vi "TEST adjust Spark Max V PID.vi"(11 "Swerve refs":cluster{"Driver":T1, "Steer":T1, "Encoder":T6}[](array[cluster])) -> ()   [LabVIEW 2023]
uses:
  <vilib>/Rock Robotics/WPI/ThirdParty/REV Robotics/REVLib/Typedef/Spark MAX Smart Motion Parameters.ctl
  <vilib>/Rock Robotics/WPI/MotorControl/WPI_MotorControlDeviceRef.ctl
  <vilib>/Rock Robotics/WPI/MotorControl/WPI_MotorControlType.ctl
  <vilib>/Rock Robotics/SystemInterfaces/DIO/FPGA_DIOPWMChannel.ctl
  <vilib>/Rock Robotics/WPI/PWM/WPI_PWMDeadband.ctl
  <vilib>/Rock Robotics/SystemInterfaces/DIO/FPGA_DIOChannel.ctl
  <vilib>/Rock Robotics/WPI/ThirdParty/Phoenix-LabVIEW/CANCoder/Controls/CTRE_Phoenix_CANcoder_DeviceRef.ctl
  <vilib>/Rock Robotics/WPI/ThirdParty/REV Robotics/REVLib/Typedef/Spark MAX Control Type.ctl
panel:
  out "Sensor Velocity":dbl
  in  "Boolean":bool
  out "Mode 2":bool caption="Mode"
  in  "motor select":i16
  in  "Velocity PID Constants":T7={"P Gain"=0.0, "I Gain"=0.0, "D Gain"=0.0, "F Gain"=0.0, "I Zone"=0.0, "Min Output"=-1.0, "Max Output"=1.0} {"Max Output" min=-1.0 max=1.0 step=0.01; "Min Output" min=-1.0 max=1.0 step=0.01; "I Zone" step=0.01; "F Gain" step=0.01; "D Gain" step=0.01; "I Gain" step=0.01; "P Gain" min=0.0 step=0.01}
  out "PID Chart":T8(graph)
  in  "Setpoint":dbl(slide) scale=-2000.0..2000.0
  in  "Smart Motion Parameters":T9={"Max Velocity"=2000.0, "Max Acceleration"=1500.0, "Minimum Velocity Output"=0.0, "Allowed Closed Loop Error"=0.0}
  in  "Mode":bool
  out "String":string="Velocity Tune"
  out "String 2":string="Smart Motion Tune"
  out "String 3":string="Tuning Instructions:\n\n0) Before using this function, you should understand from your specific mechanism the max acceleration and the max velocity. You can obtain these either by design constraints, or running in open loop mode and calculating these values.\n\n1) Set the 'Mode' switch to 'Velocity Tune'\n\n2) Tune the mechanism as you would a Velocity PID loop until the mechanism is controlled fairly well. In this mode the Setpoint slider controls the Velocity of the mechanism.\n\n3) Configure the smart motion parameters, and set the 'Mode' switch to 'Smart Motion'. In this mode, the Setpoint slider controls the Position of the mechansim. For initial tests it is recommended to keep the max velocity and max acceleration lower than the max value, and slowly increase these to the desired level.\n\n4) Test the mechanism by setting the position within the allowable range of the mechanism, and slowly increase limits until the system is working as intended."
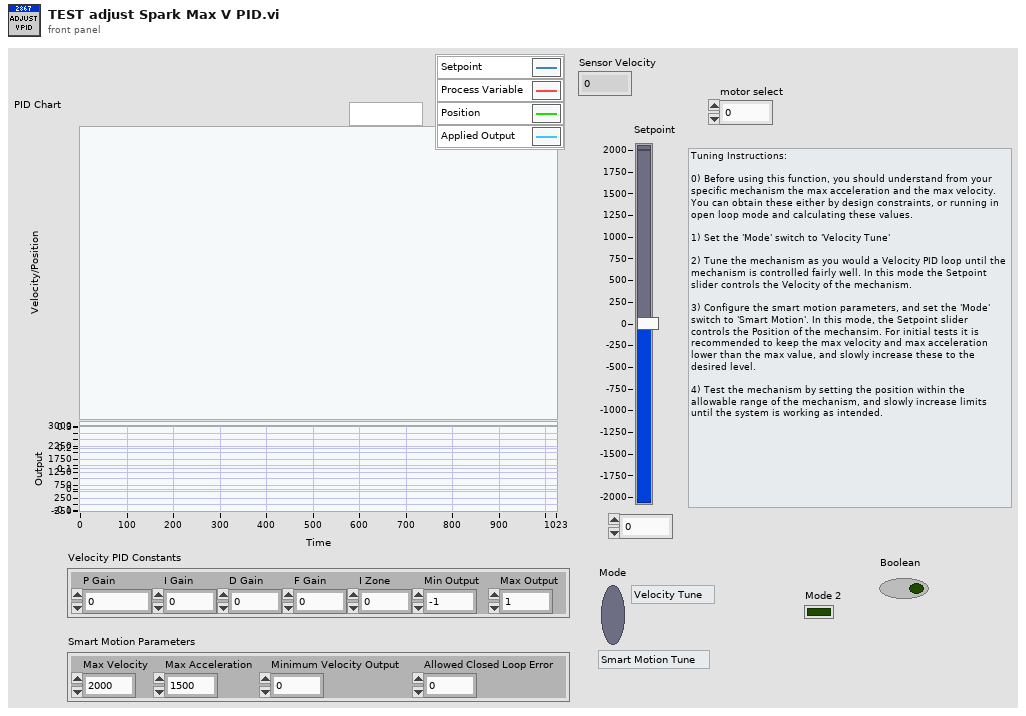
[diagram p1: front panel]
types:
  T1 = typedef "WPI_MotorControlDeviceRef.ctl" = cluster{"DeviceStatus":errorcluster, "Type":T2, "PWM":cluster{"PWM Channel":T3, "DeadBand":T4}, "CAN":cluster{"Device Number":u8, "SetOutput VI Ref":variant, "GetOutput VI Ref":variant, "Enable VI Ref":variant, "Disable VI Ref":variant, "Data":variant}, "Invert":bool, "DIO PWM":cluster{"PWM \"Enable\" Channel":T3, "DIOChannel":T5, "PWM Rate":dbl}}
  T2 = typedef "WPI_MotorControlType.ctl" = enum16{"PWM", "CAN", "DIO PWM"}
  T3 = typedef "FPGA_DIOPWMChannel.ctl" = enum8{"PWM 0", "PWM 1", "PWM 2", "PWM 3", "PWM 4", "PWM 5", "PWM 6", "PWM 7", "PWM 8", "PWM 9", "PWM MXP 0", "PWM MXP 1", "PWM MXP 2", "PWM MXP 3", "PWM MXP 4", "PWM MXP 5", "PWM MXP 6", "PWM MXP 7", "PWM MXP 8", "PWM MXP 9", "Invalid"}
  T4 = typedef "WPI_PWMDeadband.ctl" = cluster{"Name":string, "maxPositivePwm":i32, "minPositivePwm":i32, "centerPwm":i32, "maxNegativePwm":i32, "minNegativePwm":i32, "angularRange":u16}
  T5 = typedef "FPGA_DIOChannel.ctl" = enum8{"DIO 0", "DIO 1", "DIO 2", "DIO 3", "DIO 4", "DIO 5", "DIO 6", "DIO 7", "DIO 8", "DIO 9", "DIO MXP 0", "DIO MXP 1", "DIO MXP 2", "DIO MXP 3", "DIO MXP 4", "DIO MXP 5", "DIO MXP 6", "DIO MXP 7", "DIO MXP 8", "DIO MXP 9", "DIO MXP 10", "DIO MXP 11", "DIO MXP 12", "DIO MXP 13", "DIO MXP 14", "DIO MXP 15", "SPI Port CS1", "SPI Port CS2", "SPI Port CS3", "SPI Port MISO", "SPI Port MOSI", "Invalid"}
  T6 = typedef "CTRE_Phoenix_CANcoder_DeviceRef.ctl" = cluster{"DeviceStatus":errorcluster, "Device Number":u8, "Handle":u64, "UsageFrame":u32, "Library Path":path}
  T7 = cluster{"P Gain":dbl, "I Gain":dbl, "D Gain":dbl, "F Gain":dbl, "I Zone":dbl, "Min Output":dbl, "Max Output":dbl}
  T8 = cluster{"Sensor Velocity":dbl, "Setpoint":dbl, "Sensor Position":dbl, "Applied Output":dbl}
  T9 = typedef "Spark MAX Smart Motion Parameters.ctl" = cluster{"Max Velocity":dbl, "Max Acceleration":dbl, "Minimum Velocity Output":dbl, "Allowed Closed Loop Error":dbl}
  T10 = typedef "Spark MAX Control Type.ctl" = enum16{"Percent VBus", "Voltage", "Velocity", "Position", "Smart Motion", "Current", "Smart Velocity"}
  T11 = cluster{"P Gain":bool, "I Gain":bool, "D Gain":bool, "F Gain":bool, "I Zone":bool, "Min Output":bool, "Max Output":bool}
  T12 = cluster{"Max Velocity":bool, "Max Acceleration":bool, "Minimum Velocity Output":bool, "Allowed Closed Loop Error":bool}
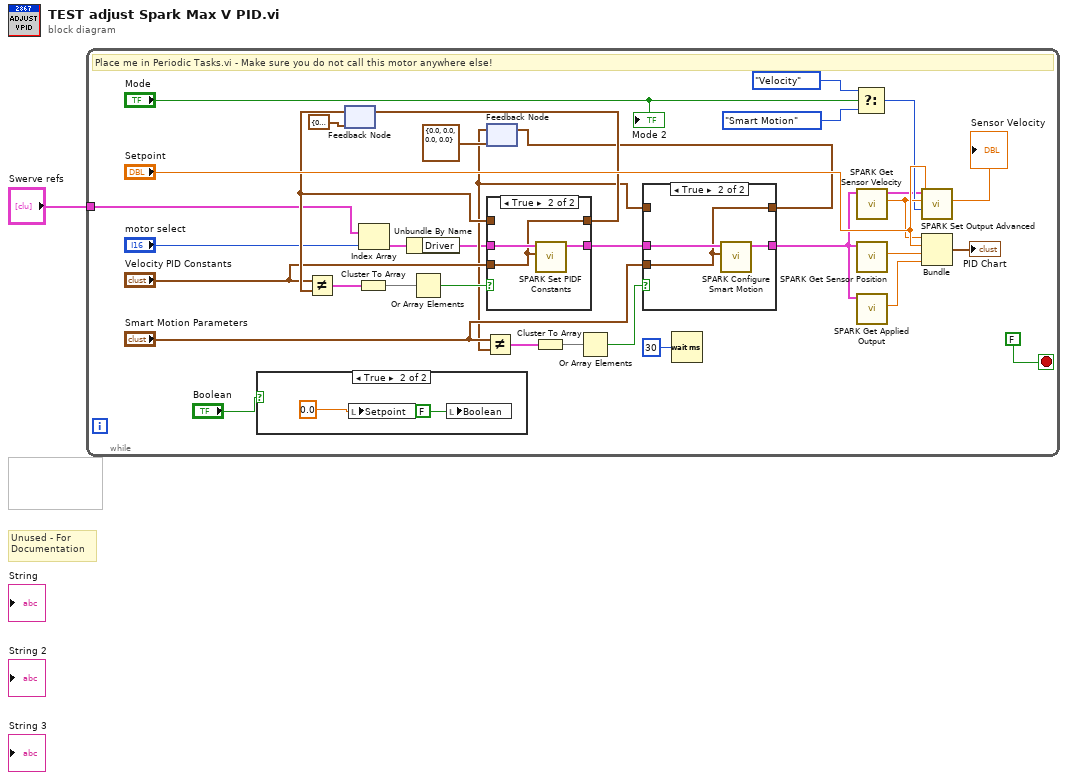
[diagram p0: block diagram]
diagram:
  # "Unused - For Documentation"
  n1 = while {
    tunnel: "Swerve refs" -> [w4]
    stop <- FALSE stop-if-true
    # "Place me in Periodic Tasks.vi - Make sure you do not call this motor anywhere else!"
    n2 = case shown="True" "Boolean" {
      frame False {
      }
      frame True {
        n3 = local write "Setpoint"(0.0 ("Setpoint")) -> ()
        n4 = local write "Boolean"(FALSE ("Boolean")) -> ()
      }
    }
    n5 = feedback #1(T7 {"P Gain"=0.0, "I Gain"=0.0, "D Gain"=0.0, "F Gain"=0.0, "I Zone"=0.0, "Min Output"=0.0, "Max Output"=0.0} ("PID Constants")) -> (w31:T7)
    n6 = Not Equal?(x="Velocity PID Constants", y=w31) -> (x != y?=w25:T11)
    n7 = Cluster To Array(cluster=w25) -> (array=w26:bool[])
    n8 = Index Array(array=w4, index="motor select") -> (element=w6:cluster{"Driver":T1, "Steer":T1, "Encoder":T6})
    n9 = Unbundle By Name(w6) -> ("Driver"=w3:T1)
    n10 = Or Array Elements(Boolean array=w26) -> (logical OR=w28:bool)
    n11 = feedback #2(T9 {"Max Velocity"=0.0, "Max Acceleration"=0.0, "Minimum Velocity Output"=0.0, "Allowed Closed Loop Error"=0.0} ("Smart Motion Parameters")) -> (w14:T9)
    n12 = Not Equal?(x="Smart Motion Parameters", y=w14) -> (x != y?=w19:T12)
    n13 = case shown="True" w28 {
      tunnel: w3 -> [w42 w46]
      tunnel: "Velocity PID Constants" -> [_ w44]
      tunnel: [w43 w44] -> w30
      tunnel: w31 -> [w43 _]
      tunnel: [w42 w45] -> w21
      frame False {
      }
      frame True {
        n14 = call <vilib>:"SPARK Set PIDF Constants.vi"("PID Constants"=w44, "MotorControlDeviceRef"=w46) -> ("MotorControlDeviceRef"=w45:T1)  [unwired: 8 in, 1 out]
      }
    }
    n15 = feedback-in #1(w30) -> ()
    n16 = Cluster To Array(cluster=w19) -> (array=w20:bool[])
    n17 = Or Array Elements(Boolean array=w20) -> (logical OR=w18:bool)
    n18 = case shown="True" w18 {
      tunnel: w21 -> [w38 w41]
      tunnel: "Smart Motion Parameters" -> [_ w39]
      tunnel: [w38 w40] -> w8
      tunnel: [w37 w39] -> w15
      tunnel: w14 -> [w37 _]
      frame False {
      }
      frame True {
        n19 = call <vilib>:"SPARK Configure Smart Motion.vi"("Smart Motion Parameters"=w39, "MotorControlDeviceRef"=w41) -> ("MotorControlDeviceRef"=w40:T1)  [unwired: 8 in, 1 out]
      }
    }
    n20 = feedback-in #2(w15) -> ()
    n21 = Wait (ms)(milliseconds to wait=u32 30) -> ()  [unwired: 1 out]
    n22 = Select(t=Spark_MAX_Control_Type."Velocity" ("Control Mode"), s="Mode", f=Spark_MAX_Control_Type."Smart Motion" ("Control Mode")) -> (s? t:f=w10:T10)
    n23 = call <vilib>:"SPARK Get Sensor Velocity.vi"("MotorControlDevRef in"=w8) -> ("Sensor Velocity"=w22:dbl, "MotorControlDevRef out"=w9:T1)  [unwired: 7 in, 2 out]
    "Sensor Velocity" <- w22
    n24 = call <vilib>:"SPARK Get Sensor Position.vi"("MotorControlDevRef in"=w8) -> ("Sensor Position"=w34:dbl)  [unwired: 7 in, 3 out]
    n25 = call <vilib>:"SPARK Get Applied Output.vi"("MotorControlDevRef in"=w8) -> ("Applied Output"=w7:dbl)  [unwired: 7 in, 3 out]
    n26 = call <vilib>:"SPARK Set Output Advanced.vi"("Control Mode"=w10, "Setpoint"="Setpoint", "MotorControlDevRef"=w9) -> ()  [unwired: 7 in, 2 out]
    n27 = Bundle("Sensor Velocity"=w22, "Setpoint"="Setpoint", "Sensor Position"=w34, "Applied Output"=w7) -> (→"PID Chart":T8)  [unwired: 1 in]
    "Mode 2" <- "Mode"
  }
